vi "Assignment W5.vi"() -> ()   [LabVIEW 2023]
uses:
  Khoa A5 C1.ctl
panel:
  in  "stop":bool
  out "Color 2":string
  out "Color 1":string
  out "Traffic Light 2":bool[](array[boolean])
  out "Traffic Light 1":bool[](array[boolean])
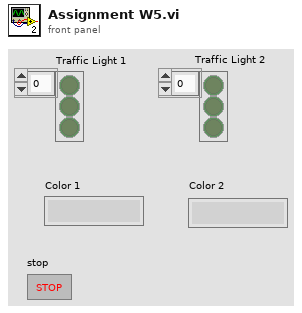
[diagram p1: front panel]
types:
  T1 = typedef "Khoa A5 C1.ctl" = enum16{"Idle", "Red/Green", "Red/Amber", "Green/Red", "Amber/Red"}
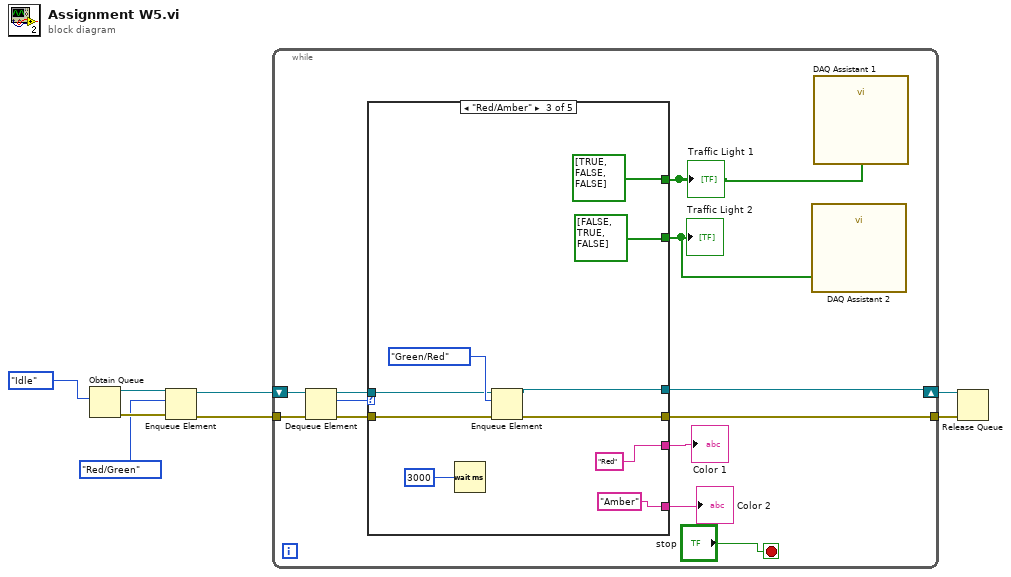
[diagram p0: block diagram]
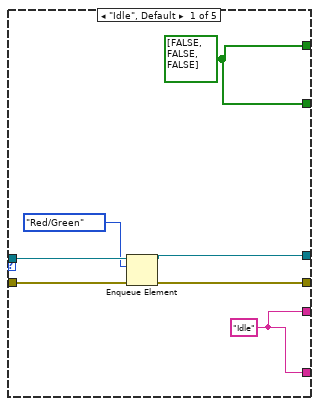
[diagram p2: hidden frame]
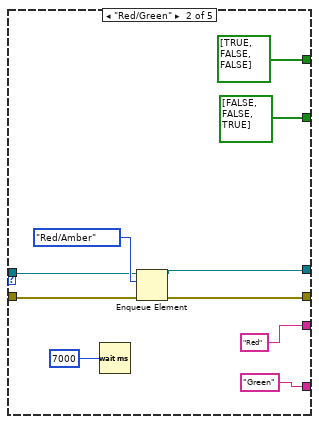
[diagram p3: hidden frame]
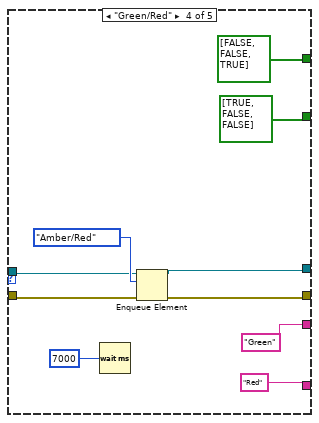
[diagram p4: hidden frame]
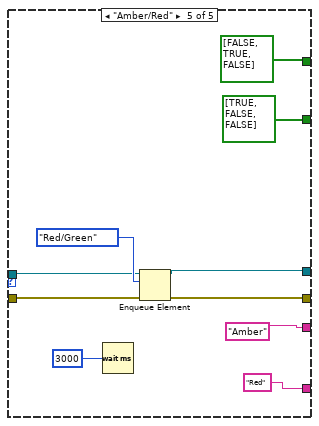
[diagram p5: hidden frame]
diagram:
  n1 = Obtain Queue(element data type=Khoa_A5_C1."Idle") -> (queue out=w7:refnum<queue>, error out=w5:errorcluster)  [unwired: 4 in, 1 out]
  n2 = Enqueue Element(queue=w7, element=Khoa_A5_C1."Red/Green", error in (no error)=w5) -> (queue out=w6:refnum<queue>, error out=w4:errorcluster)  [unwired: 1 in, 1 out]
  n3 = while {
    shift-right: [w15] -> w2
    shift-left: w6 -> [w19]
    tunnel: w4 -> [w20]
    tunnel: [w14] -> w1
    stop <- "stop" stop-if-true
    n4 = Dequeue Element(queue=w19, error in (no error)=w20) -> (queue out=w18:refnum<queue>, element=w16:T1, error out=w17:errorcluster)  [unwired: 1 in, 1 out]
    n5 = case shown="\"Red/Amber\"" w16 {
      tunnel: w18 -> [w27 w36 w45 w55 w65]
      tunnel: w17 -> [w25 w35 w44 w54 w64]
      tunnel: [w26 w34 w43 w53 w63] -> w15
      tunnel: [w24 w33 w42 w52 w62] -> w14
      tunnel: [w22 "Red" "Red" "Green" "Amber"] -> w13
      tunnel: [w22 "Green" "Amber" "Red" "Red"] -> w12
      tunnel: [w21 bool[] [TRUE, FALSE, FALSE] bool[] [TRUE, FALSE, FALSE] bool[] [FALSE, FALSE, TRUE] bool[] [FALSE, TRUE, FALSE]] -> w9
      tunnel: [w21 bool[] [FALSE, FALSE, TRUE] bool[] [FALSE, TRUE, FALSE] bool[] [TRUE, FALSE, FALSE] bool[] [TRUE, FALSE, FALSE]] -> w10
      frame "Idle", Default {
        w21 = bool[] [FALSE, FALSE, FALSE]
        w22 = "Idle"
        n6 = Enqueue Element(queue=w27, element=Khoa_A5_C1."Red/Green", error in (no error)=w25) -> (queue out=w26:refnum<queue>, error out=w24:errorcluster)  [unwired: 1 in, 1 out]
      }
      frame "Red/Green" {
        n7 = Wait (ms)(milliseconds to wait=7000) -> ()  [unwired: 1 out]
        n8 = Enqueue Element(queue=w36, element=Khoa_A5_C1."Red/Amber", error in (no error)=w35) -> (queue out=w34:refnum<queue>, error out=w33:errorcluster)  [unwired: 1 in, 1 out]
      }
      frame "Red/Amber" {
        n9 = Wait (ms)(milliseconds to wait=3000) -> ()  [unwired: 1 out]
        n10 = Enqueue Element(queue=w45, element=Khoa_A5_C1."Green/Red", error in (no error)=w44) -> (queue out=w43:refnum<queue>, error out=w42:errorcluster)  [unwired: 1 in, 1 out]
      }
      frame "Green/Red" {
        n11 = Wait (ms)(milliseconds to wait=7000) -> ()  [unwired: 1 out]
        n12 = Enqueue Element(queue=w55, element=Khoa_A5_C1."Amber/Red", error in (no error)=w54) -> (queue out=w53:refnum<queue>, error out=w52:errorcluster)  [unwired: 1 in, 1 out]
      }
      frame "Amber/Red" {
        n13 = Wait (ms)(milliseconds to wait=3000) -> ()  [unwired: 1 out]
        n14 = Enqueue Element(queue=w65, element=Khoa_A5_C1."Red/Green", error in (no error)=w64) -> (queue out=w63:refnum<queue>, error out=w62:errorcluster)  [unwired: 1 in, 1 out]
      }
    }
    "Traffic Light 2" <- w10
    "Traffic Light 1" <- w9
    "Color 2" <- w12
    "Color 1" <- w13
    n15 = call "DAQ Assistant 2"("data"=w10) -> ()  [unwired: 17 in, 2 out]
    n16 = call "DAQ Assistant 1"("data"=w9) -> ()  [unwired: 17 in, 2 out]
  }
  n17 = Release Queue(queue=w2, error in (no error)=w1) -> ()  [unwired: 1 in, 3 out]
